vi "Send Add View.vi"(5 "Paused (F)":bool, 6 "Receive Only (F)":bool, 7 "Priority":T1=enum."Normal" caption="Message Priority (Normal)", 8 "error in (no error)":errorcluster, 9 "Exclude From Broadcast (F)":bool, 10 "View Actor":refnum<class "View.lvclass">, 11 "Message Enqueuer in":refnum<class "Message Enqueuer.lvclass">) -> (0 "error out":errorcluster, 3 "Message Enqueuer out":refnum<class "Message Enqueuer.lvclass">)   [LabVIEW 2023, in "MVC Actors.lvlib" / "Add View Msg.lvclass"]
doc: "Sends the <b>MVC Actors.lvlib:Add View Msg.lvclass</b> message.\n\nThis message will call <b>Add View.vi</b> on the <b>MVC Actors.lvlib:Controller.lvclass</b> actor.\n\n<b>Add View.vi Description</b>\nStarts a View Actor with following settings:\n\n<b>Exclude From Broadcast</b>: message originating form another view will not be broadcasted to the view being cosidered\n<b>Paused</b>: the view will not send events and will not receive them anymore\n<b>Receive only</b>: The view will receive events but not send any"
uses:
  Add View Msg.lvclass
  Add View Msg.lvclass/Add View Msg.ctl
  <vilib>/ActorFramework/Message Enqueuer/Message Enqueuer.lvclass
  C:/Program Files/National Instruments/LabVIEW 2023/vi.lib/ActorFramework/Message/Message.lvclass
  C:/Projects/Shared Libraries/Event Actors/Controller Messages/Add View Msg/Add View Msg.lvclass
  <vilib>/ActorFramework/Message Enqueuer/Message Priority.ctl
  View/View.lvclass
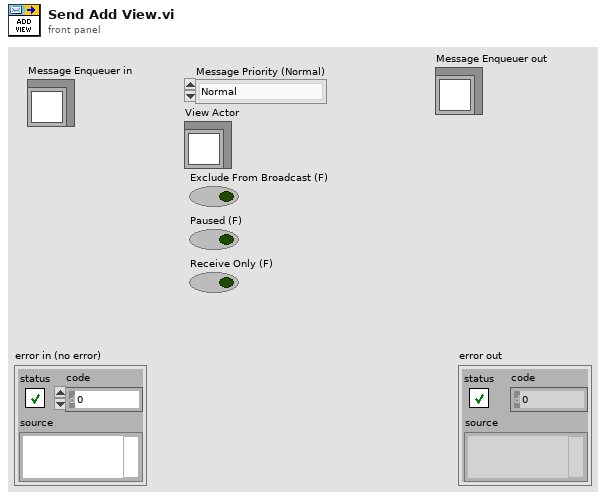
[diagram p1: front panel]
types:
  T1 = typedef "Actor Framework.lvlib/Message Enqueuer.lvclass/Message Priority.ctl" = enum16{"Low", "Normal", "High"}
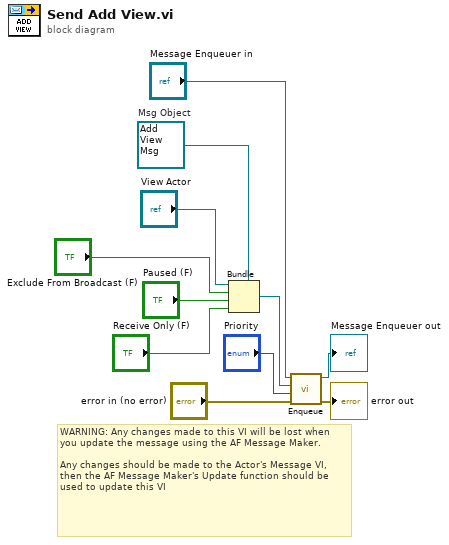
[diagram p0: block diagram]
diagram:
  w7 = refnum<class "Add View Msg.lvclass"> refnum  # Msg Object
  # "WARNING: Any changes made to this VI will be lost when you update the message using the AF Message Maker.\n\nAny changes should be made to the Actor's Message VI, then the AF Message Maker's Update function should be used to update this VI"
  n1 = Bundle(cluster=w7, "View Actor", "Exclude From Broadcast (F)", "Paused (F)", "Receive Only (F)") -> (w2:refnum<class "Add View Msg.lvclass">)
  n2 = call <vilib>:"Enqueue.vi"("error in (no error)"="error in (no error)", "Message Priority (Normal)"="Priority", "Message"=w2, "Message Enqueuer in"="Message Enqueuer in") -> ("error out"=→"error out":errorcluster, "Message Enqueuer out"=→"Message Enqueuer out":refnum<class "Message Enqueuer.lvclass">)  [unwired: 6 in]
